vi "Request Serial Number.vi"(8 "error in (no error)":errorcluster, 11 "Serial Number":string) -> (0 "error out":errorcluster, 2 "Serial Number Out":string)   [LabVIEW 2015]
panel:
  in  "OK Button":bool
  out "Test Sequence":i32(listbox)=-2
  # "Scan Serial Number"
  # "Please scan the serial number and copy and paste it into the box\nCharacter Limit - 8"
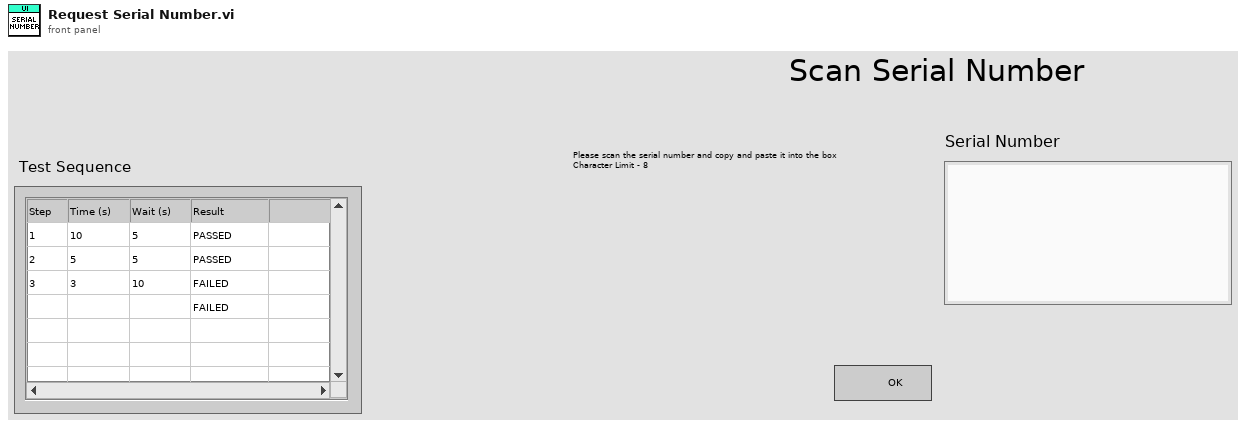
[diagram p1: front panel]
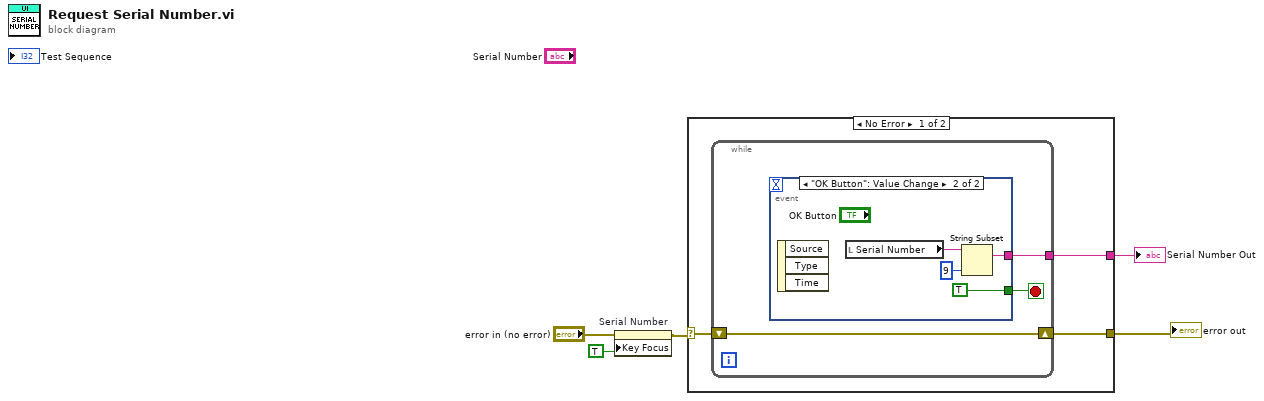
[diagram p0: block diagram]
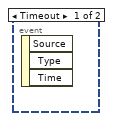
[diagram p2: hidden frame]
diagram:
  n1 = property on="Serial Number" class="Str"(error in="error in (no error)", "Key Focus"=TRUE) -> (error out=w1:errorcluster)  [unwired: 1 in, 1 out]
  n2 = case shown="No Error" w1 {
    selector: w1 -> [w7 w16]
    tunnel: [w8 _] -> w5
    tunnel: [w6 w16] -> w4
    frame No Error {
      n3 = while {
        tunnel: [w10] -> w8
        shift-right: [w9] -> w6
        shift-left: w7 -> [w9]
        stop <- w11 stop-if-true
        n4 = event shown="[1] \"OK Button\": Value Change" {
          selector: _ -> [_ _]
          dyn-events: _ -> [_ _]
          timeout: _ -> [_ _]
          tunnel: [_ TRUE] -> w11
          tunnel: [_ w12] -> w10
          event Timeout {
            n5 = event-data() -> ()  [unwired: 1 in, 3 out]
          }
          event "OK Button": Value Change {
            n6 = event-data() -> ()  [unwired: 1 in, 3 out]
            n7 = local read "Serial Number"() -> (w14:string)
            n8 = String Subset(string=w14, length (rest)=9 ("length (rest)")) -> (substring=w12:string)  [unwired: 1 in]
          }
        }
      }
    }
    frame Error {
    }
  }
  "error out" <- w4
  "Serial Number Out" <- w5
